vi "HistogramCalc.vi"(8 "error in (no error)":errorcluster, 9 "Offline":bool, 10 "Diagnostic Check Image":T1, 11 "File Path":path) -> (0 "error out":errorcluster, 2 "Image Out":T1, 3 "Histogram Report":T2 {"Standard  Variation" format="%.2f"; "Mean Value" format="%.2f"; "Interval Width" format="%.2f"; "Starting Value" format="%.2f"; "Maximal Value" format="%.2f"; "Minimal Value" format="%.2f"})   [LabVIEW 2019]
uses:
  <vilib>/vision/Image Controls.llb/IMAQ Image.ctl
  <vilib>/vision/NI_Vision_Development_Module.lvlib
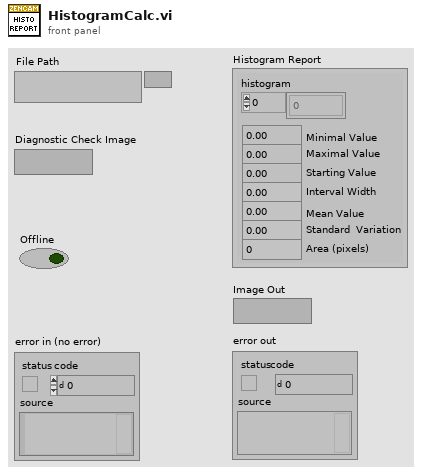
[diagram p1: front panel]
types:
  T1 = typedef "IMAQ Image.ctl" = refnum<image>
  T2 = cluster{"histogram":u32[], "Minimal Value":sgl, "Maximal Value":sgl, "Starting Value":sgl, "Interval Width":sgl, "Mean Value":sgl, "Standard  Variation":sgl, "Area (pixels)":i32}
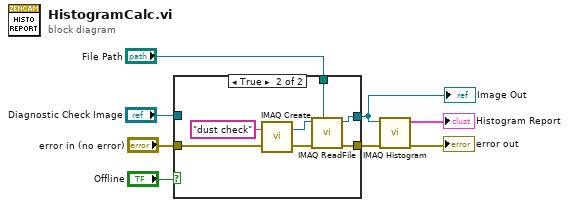
[diagram p0: block diagram]
diagram:
  n1 = case shown="True" "Offline" {
    tunnel: "File Path" -> [_ w17]
    tunnel: [w10 w16] -> w7
    tunnel: "error in (no error)" -> [w10 w15]
    tunnel: [w9 w14] -> w3
    tunnel: "Diagnostic Check Image" -> [w9 _]
    frame False {
    }
    frame True {
      n2 = call "IMAQ Create"("Image Name"="dust check", "error in (no error)"=w15) -> ("New Image"=w12:T1, "error out"=w13:errorcluster)  [unwired: 3 in]
      n3 = call "IMAQ ReadFile"("File Path"=w17, "error in (no error)"=w13, "Image"=w12) -> ("error out"=w16:errorcluster, "Image Out"=w14:T1)  [unwired: 4 in, 3 out]
    }
  }
  "Image Out" <- w3
  n4 = call "IMAQ Histogram"("error in (no error)"=w7, "Image"=w3) -> ("error out"=→"error out":errorcluster, "Histogram Report"=→"Histogram Report":T2)  [unwired: 8 in]
